vi "SerialFWDR.vi"(8 "error in (no error)":errorcluster, 9 "Delay Time (s)":dbl=1.0, 10 "CommandString":string, 11 "VISA Refnum in":refnum<visa-resource-name>) -> (0 "error out":errorcluster, 2 "trimmed string":string, 3 "VISA Refnum out":refnum<visa-resource-name>)   [LabVIEW 2017]
uses:
  <vilib>/Instr/_visa.llb/VISA Flush IO Buffer Mask.ctl
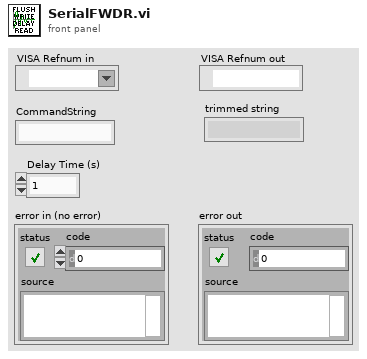
[diagram p1: front panel]
types:
  T1 = typedef "VISA Flush IO Buffer Mask.ctl" = u16
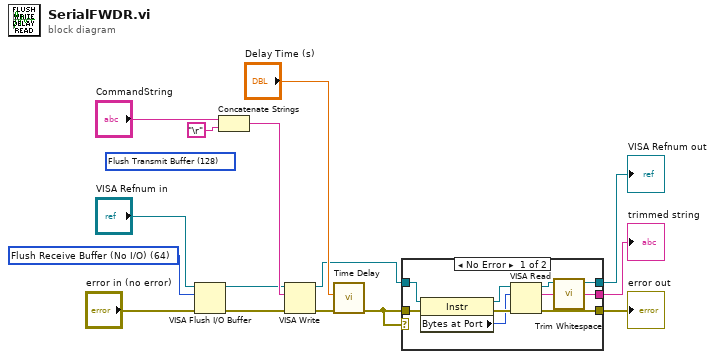
[diagram p0: block diagram]
diagram:
  w8 = T1 64 items=["Flush Receive Buffer"=16, "Write Transmit Buffer to Device"=32, "Flush Receive Buffer (No I/O)"=64, "Flush Transmit Buffer"=128] ("Mask")
  (unwired) T1 128 items=["Flush Receive Buffer"=16, "Write Transmit Buffer to Device"=32, "Flush Receive Buffer (No I/O)"=64, "Flush Transmit Buffer"=128] ("Mask")
  n1 = VISA Flush I/O Buffer(VISA resource name="VISA Refnum in", mask (16)=w8, error in (no error)="error in (no error)") -> (VISA resource name out=w2:refnum<visa-resource-name>, error out=w1:errorcluster)
  n2 = Concatenate Strings("CommandString", "\r") -> (w11:string)
  n3 = VISA Write(VISA resource name=w2, write buffer=w11, error in (no error)=w1) -> (VISA resource name out=w7:refnum<visa-resource-name>, error out=w9:errorcluster)  [unwired: 1 out]
  n4 = call "Time Delay"("error in (no error)"=w9, "Delay Time (s)"="Delay Time (s)") -> ("error out"=w3:errorcluster)  [unwired: 9 in]
  n5 = case shown="No Error" w3 {
    tunnel: w3 -> [w20 w26]
    tunnel: [w23 w26] -> w6
    tunnel: [w22 w25] -> w4
    tunnel: w7 -> [w17 w25]
    tunnel: [w16 _] -> w5
    frame No Error {
      n6 = property class="Instr"(reference=w17, error in=w20) -> (reference out=w21:refnum<visa-resource-name>, error out=w19:errorcluster, "Bytes at Port"=w18:u32)
      n7 = VISA Read(VISA resource name=w21, byte count=w18, error in (no error)=w19) -> (VISA resource name out=w22:refnum<visa-resource-name>, read buffer=w24:string, error out=w23:errorcluster)  [unwired: 1 out]
      n8 = call <vilib>:"Trim Whitespace.vi"("string"=w24) -> ("trimmed string"=w16:string)  [unwired: 1 in]
    }
    frame Error {
    }
  }
  "VISA Refnum out" <- w4
  "error out" <- w6
  "trimmed string" <- w5
